vi "Initialize.vi"(8 "error in":errorcluster, 10 "shared resources":refnum<class "Shared Resources.lvclass">, 11 "Ballard ARINC-429 Rx Execution Unit in":refnum<class "Rx Execution Unit.lvclass">) -> (0 "error out":errorcluster, 3 "Ballard ARINC-429 Rx Execution Unit out":refnum<class "Rx Execution Unit.lvclass">)   [LabVIEW 2020, in "Ballard ARINC 429 Engine.lvlib" / "Implementation.lvlib" / "Rx Execution Unit.lvclass"]
uses:
  Rx Execution Unit.lvclass
  C:/Users/nitest/Desktop/niveristand-ballard-arinc429-custom-device/Source/Custom Device Support/Engine/Implementation/Execution Unit/Execution Unit.lvclass
  Interfaces/Shared Resources/Shared Resources.lvclass
  Shared Resources/Shared Resources.lvclass
  Shared Resources/Shared Resources.lvclass/Shared Resources.ctl
  Execution Unit/Execution Unit.lvclass/Execution Unit.ctl
  Rx Execution Unit.lvclass/Rx Execution Unit.ctl
  Custom Device/Custom Device.lvlib
  Execution Unit/Execution Unit.lvclass
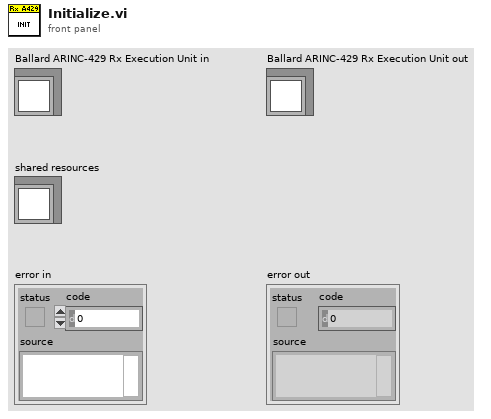
[diagram p1: front panel]
types:
  T1 = typedef "Ballard ARINC 429 Engine.lvlib/Custom Device.lvlib/Hardware Handles.ctl" = cluster{"core handle":u64, "core reader handle":u64, "channel handles":u64[]}
  T2 = typedef "RT Hardware Channel Settings.ctl" = cluster{"channel #":u16, "channel handle":u64, "labels settings for RT":T3[]}
  T3 = typedef "RT Label Settings.ctl" = cluster{"Name":string, "xmlName":string, "label":T4, "transfer period":u32, "SDI_Enabled":bool, "SDI":u8, "parameter driver data":T5, "transfer type":T9, "has timestamp?":bool, "Label Disable/Trigger Channel Reference":T8, "Message Handle":u64, "Initialized?":bool, "Word Initial Raw Value":u32, "Label Timestamp Channel Data Reference":T10, "disabled":bool}
  T4 = typedef "Label.ctl" = u8
  T5 = typedef "RT Parameters.ctl" = cluster{"parameter definitions":T6[], "Tx parameter refs":T8[]}
  T6 = typedef "Parameter Definition.ctl" = cluster{"start index":i32, "size":i32, "encoding":T7, "signed":bool, "scale multiplier":dbl, "scale offset":dbl}
  T7 = typedef "Encoding and Decoding.lvlib/Encoding.ctl" = enum16{"BNR", "BCD", "Discrete"}
  T8 = typedef "Custom Device API.lvlib/Custom Device Item Ref.ctl" = u64
  T9 = typedef "Transfer Type.ctl" = enum16{"Scheduled", "Acyclic", "Block", "Strobe"}
  T10 = typedef "Custom Device API.lvlib/Data Reference.ctl" = i32
  T11 = typedef "Map of Identifiers to Indexes.ctl" = map{u32, cluster{"channel index":i32, "label index":i32, "start index":i32, "parameters":i32, "timestamp index":i32}}
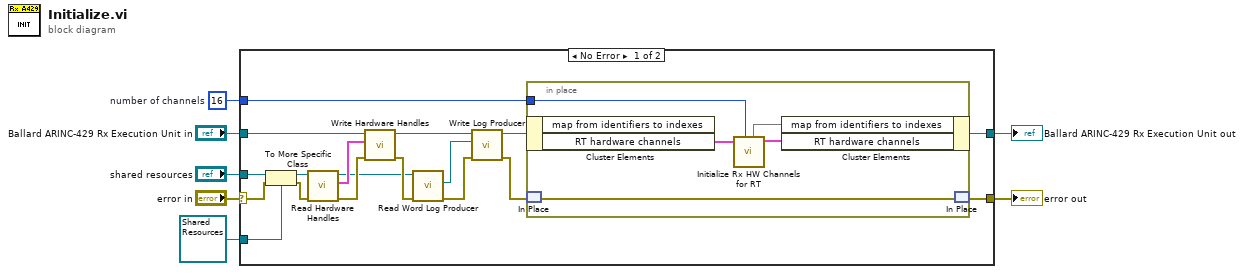
[diagram p0: block diagram]
diagram:
  w5 = 16  # number of channels
  n1 = case shown="No Error" "error in" {
    selector: "error in" -> [w14 w32]
    tunnel: "Ballard ARINC-429 Rx Execution Unit in" -> [w22 w31]
    tunnel: [w25 w31] -> w6
    tunnel: w5 -> [w24 _]
    tunnel: [w18 w32] -> w4
    tunnel: "shared resources" -> [w16 _]
    tunnel: refnum<class "Shared Resources.lvclass"> refnum ("Ballard ARINC-429 shared resources in") -> [w17 _]
    frame No Error {
      n2 = To More Specific Class(target class=w17, reference=w16, error in=w14) -> (specific class reference=w15:refnum<class "Shared Resources.lvclass">, error out=w13:errorcluster)
      n3 = call "Read Hardware Handles.vi"("error in"=w13, "Ballard ARINC-429 shared resources in"=w15) -> ("error out"=w21:errorcluster, "hardware handles"=w20:T1, "Ballard ARINC-429 shared resources out"=w12:refnum<class "Shared Resources.lvclass">)  [unwired: 7 in]
      n4 = call "Write Hardware Handles.vi"("error in"=w21, "hardware handles"=w20, "Ballard ARINC-429 Execution Unit in"=w22) -> ("error out"=w19:errorcluster, "Ballard ARINC-429 Execution Unit out"=w23:refnum<class "Rx Execution Unit.lvclass">)  [unwired: 7 in]
      n5 = call-dynamic "Read Word Log Producer.vi"("error in (no error)"=w19, "Shared Resources in"=w12) -> ("error out"=w10:errorcluster, "Communication Bus Template Interfaces:Implementation.lvlib:Logging.lvlib:Word Log Producer.lvclass"=w8:refnum<class "Log Producer.lvclass">)  [unwired: 7 in, 1 out]
      n6 = call-dynamic "Write Log Producer.vi"("error in (no error)"=w10, "Log Producer"=w8, "Rx Execution Unit in"=w23) -> ("error out"=w9:errorcluster, "Rx Execution Unit out"=w11:refnum<class "Rx Execution Unit.lvclass">)  [unwired: 7 in]
      n7 = in-place {
        in-place-border: w24 -> [w30]
        n8 = in-place-cluster #1(w11) -> ("RT hardware channels"=w27:T2[])  [unwired: 1 out]
        n9 = in-place-match #2(w9) -> (w29:errorcluster)
        n10 = call "Initialize Rx HW Channels for RT.vi"("number of channels"=w30, "Rx Channels In"=w27) -> ("Rx Channels Out"=w28:T2[], "map from identifiers to indexes"=w26:T11)  [unwired: 6 in]
        n11 = in-place-cluster #1("map from identifiers to indexes"=w26, "RT hardware channels"=w28) -> (w25:refnum<class "Rx Execution Unit.lvclass">)
        n12 = in-place-match #2(w29) -> (w18:errorcluster)
      }
    }
    frame Error {
    }
  }
  "error out" <- w4
  "Ballard ARINC-429 Rx Execution Unit out" <- w6
